vi "hamamatsuRead.vi"   [LabVIEW 2017]
uses:
  globalDevices.vi
  globalUtilities.vi
types:
  T1 = enum16{"open", "replace", "create", "open or create", "replace or create", "replace or create with confirmation"}
  T2 = enum16{"big-endian, network order", "native, host order", "little-endian"}
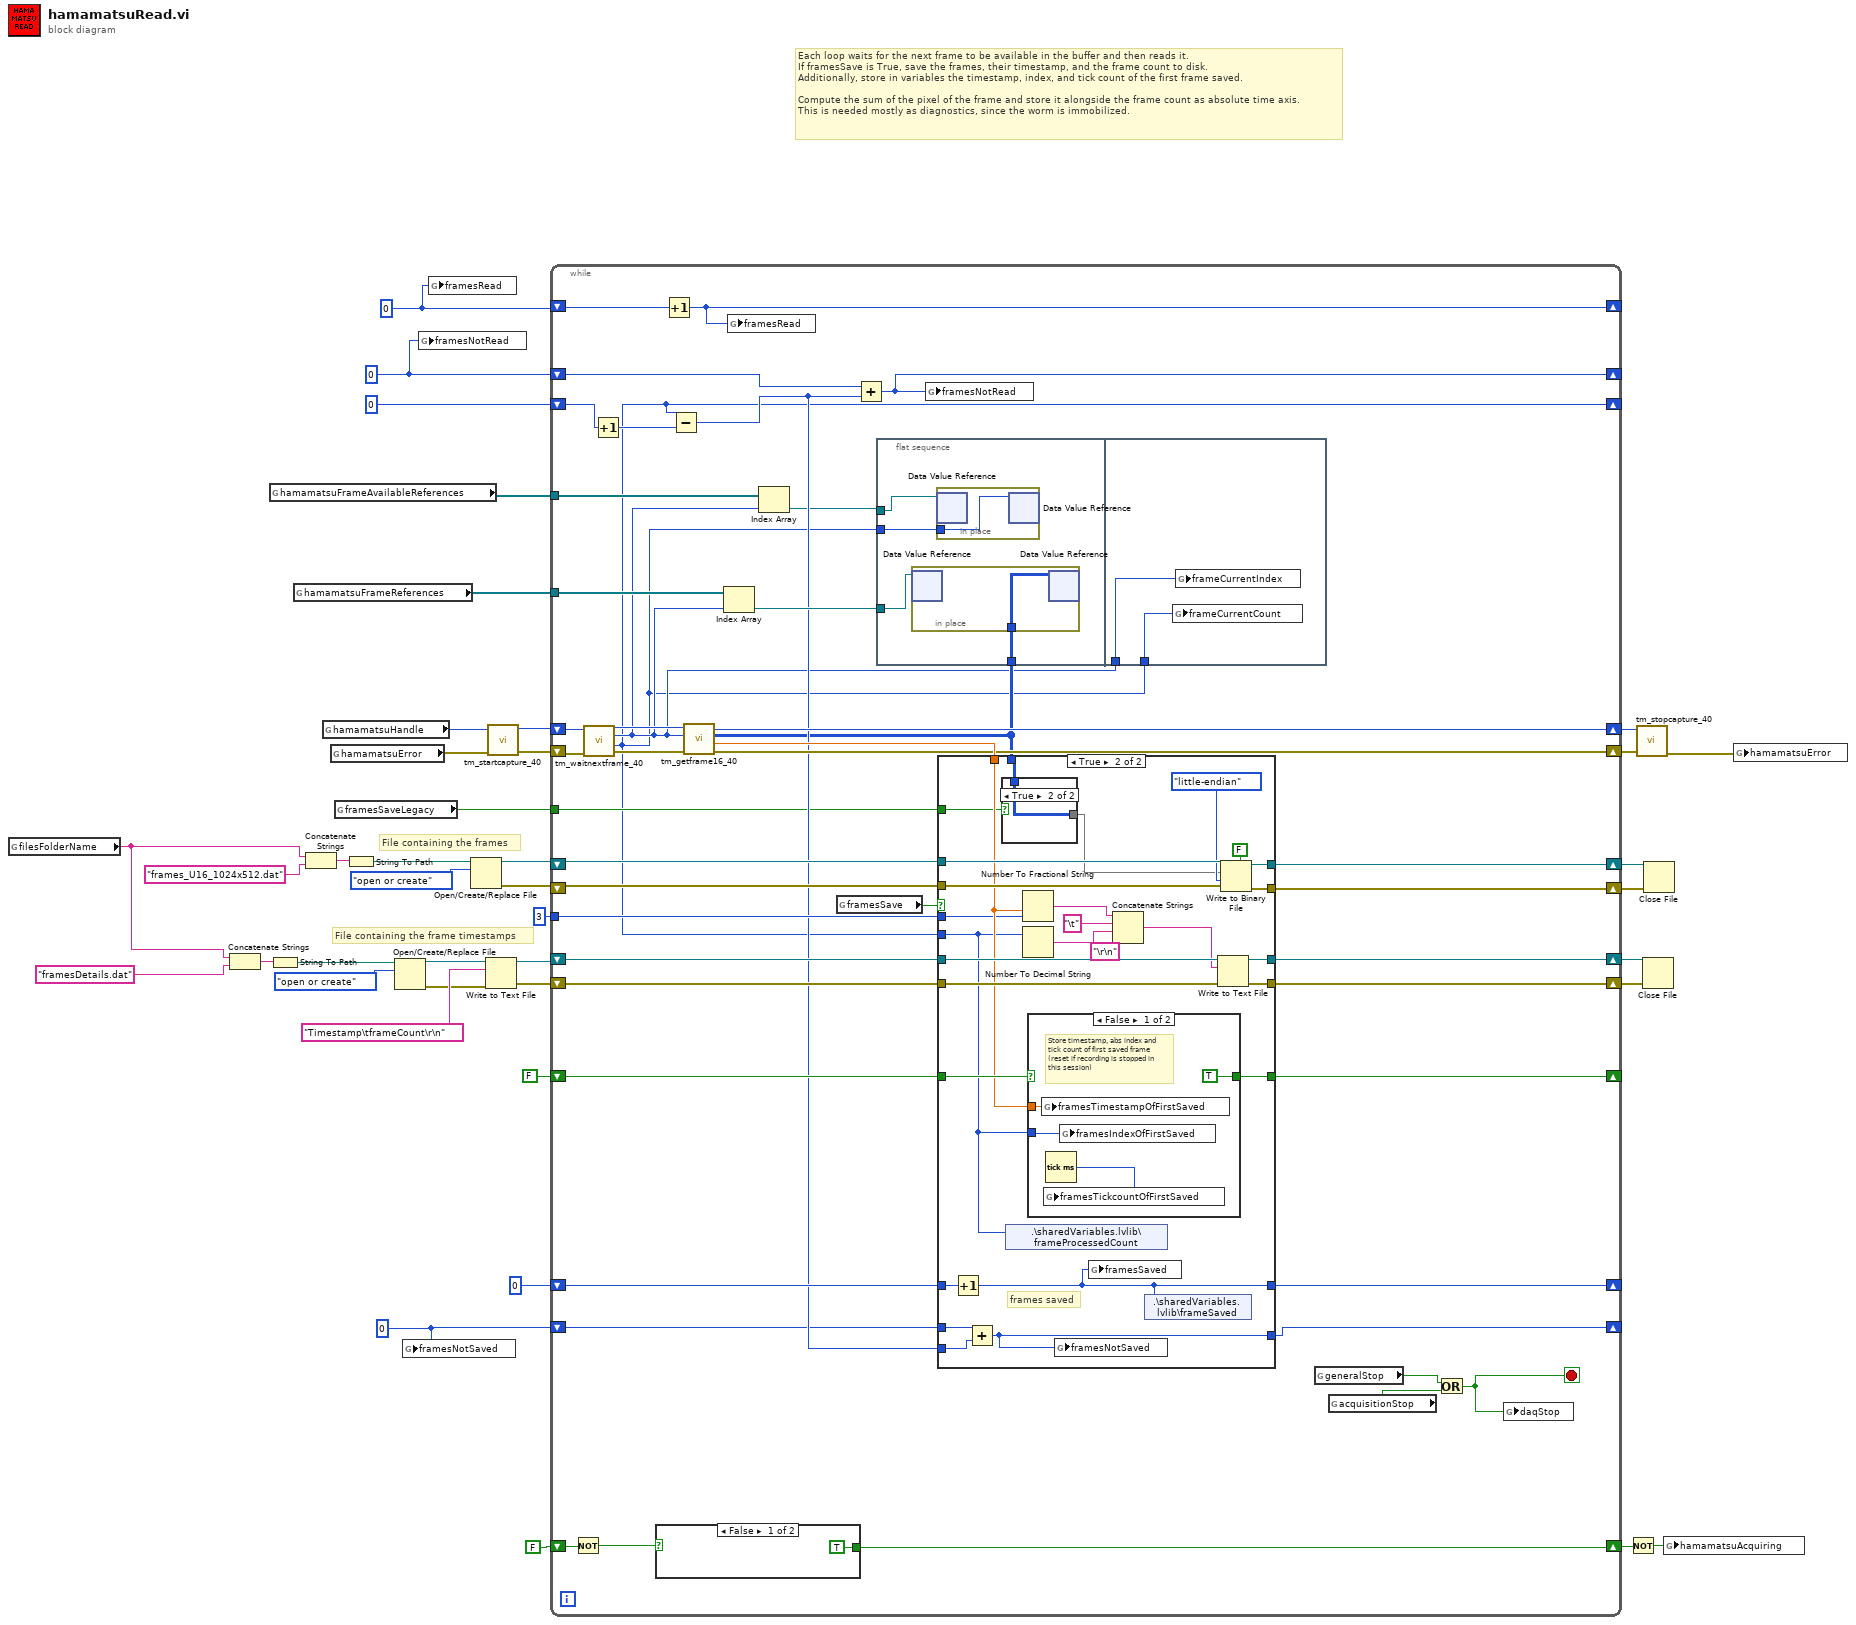
[diagram p0: block diagram]
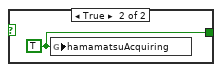
[diagram p2: hidden frame]
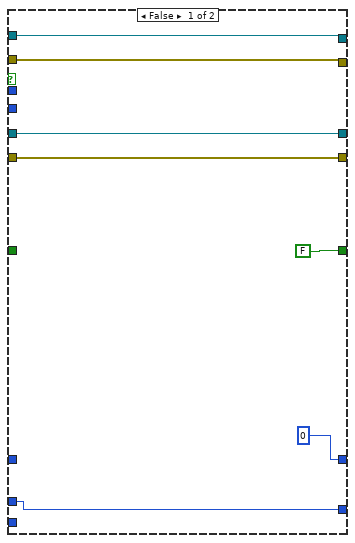
[diagram p3: hidden frame]
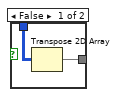
[diagram p4: hidden frame]
diagram:
  w1 = u32 0 ("framesRead")
  w5 = 0
  w2 = 0
  # "Each loop waits for the next frame to be available in the buffer and then reads it.\nIf framesSave is True, save the frames, their timestamp, and the frame count to disk.\nAdditionally, store in variables the timestamp, index, and tick count of the first frame saved.\n\nCompute the sum of the pixel of the frame and store it alongside the frame count as absolute time axis.\nThis is needed mostly as diagnostics, since the worm is immobilized."
  # "File containing the frame timestamps"
  # "File containing the frames"
  n1 = global read "globalUtilities.vi" "filesFolderName"() -> (w23:string)
  n2 = Concatenate Strings(w23, "framesDetails.dat") -> (w33:string)
  n3 = global read "globalDevices.vi" "hamamatsuFrameAvailableReferences"() -> (w6:refnum<data-value>[])
  n4 = String To Path(string=w33) -> (path=w34:path)
  n5 = global read "globalDevices.vi" "hamamatsuFrameReferences"() -> (w10:refnum<data-value>[])
  n6 = Concatenate Strings(w23, "frames_U16_1024x512.dat") -> (w38:string)
  n7 = global read "globalDevices.vi" "hamamatsuHandle"() -> (w19:u32)
  n8 = global read "globalDevices.vi" "hamamatsuError"() -> (w20:errorcluster)
  n9 = global read "globalUtilities.vi" "framesSaveLegacy"() -> (w7:bool)
  n10 = String To Path(string=w38) -> (path=w37:path)
  n11 = Open/Create/Replace File(file path (use dialog)=w34, operation (0:open)=T1."open or create") -> (refnum out=w28:refnum<file>, error out=w26:errorcluster)  [unwired: 4 in, 1 out]
  n12 = global write "globalUtilities.vi" "framesNotSaved"(w5) -> ()
  n13 = global write "globalUtilities.vi" "framesNotRead"(w2) -> ()
  n14 = global write "globalUtilities.vi" "framesRead"(w1) -> ()
  n15 = Open/Create/Replace File(file path (use dialog)=w37, operation (0:open)=T1."open or create") -> (refnum out=w36:refnum<file>, error out=w30:errorcluster)  [unwired: 4 in, 1 out]
  n16 = Write to Text File(file (use dialog)=w28, text="Timestamp\tframeCount\r\n", error in=w26) -> (refnum out=w25:refnum<file>, error out=w24:errorcluster)  [unwired: 1 in, 1 out]
  n17 = call <userlib>:"tm_startcapture_40.vi"("error in (no error)"=w20, "Handle in"=w19) -> ("error out"=w21:errorcluster, "Handle out"=w22:u32)  [unwired: 8 in]
  n18 = while {
    shift-right: [w71] -> _
    shift-left: FALSE -> [w72]
    shift-right: [w77] -> w13
    shift-left: w24 -> [w78]
    shift-right: [w75] -> w15
    shift-left: w30 -> [w76]
    tunnel: i16 3 ("precision (6)") -> [w70]
    shift-right: [w69] -> w18
    shift-left: w21 -> [w83]
    shift-right: [w67] -> _
    shift-left: u32 0 -> [w68]
    shift-right: [w66] -> w17
    shift-left: w22 -> [w84]
    shift-right: [w64] -> w12
    shift-left: w25 -> [w79]
    shift-right: [w65] -> w14
    shift-left: w36 -> [w80]
    tunnel: w10 -> [w60]
    shift-right: [w43] -> _
    shift-left: 0 -> [w58]
    shift-right: [w56] -> _
    shift-left: w2 -> [w57]
    shift-right: [w53] -> _
    shift-left: w5 -> [w54]
    tunnel: w7 -> [w52]
    tunnel: w6 -> [w48]
    shift-right: [w45] -> w3
    shift-left: FALSE -> [w47]
    shift-right: [w41] -> _
    shift-left: w1 -> [w42]
    stop <- w61 stop-if-true
    n19 = Not(x=w47) -> (.not. x?=w46:bool)
    n20 = call <userlib>:"tm_waitnextframe_40.vi"("error in (no error)"=w83, "Handle in"=w84) -> ("error out"=w82:errorcluster, "Frame Count"=w43:i32, "Frame Index"=w49:i32, "Handle out"=w81:u32)  [unwired: 6 in]
    n21 = Increment(x=w58) -> (x+1=w51:i32)
    n22 = case shown="False" w46 {
      tunnel: [TRUE w86] -> w45
      frame False {
      }
      frame True {
        w86 = TRUE ("hamamatsuAcquiring")
        n23 = global write "globalUtilities.vi" "hamamatsuAcquiring"(w86) -> ()
      }
    }
    n24 = Increment(x=w42) -> (x+1=w41:u32)
    n25 = Subtract(x=w43, y=w51) -> (x-y=w55:i32)
    n26 = call <userlib>:"tm_getframe16_40.vi"("error in (no error)"=w82, "Frame Index"=w49, "Handle in"=w81) -> ("error out"=w69:errorcluster, "Timestamp"=w73:dbl, "Data"=w50:u16[][], "Handle out"=w66:u32)  [unwired: 5 in]
    n27 = Index Array(array=w60, index=w49) -> (element=w59:refnum<data-value>)
    n28 = global write "globalUtilities.vi" "framesRead"(w41) -> ()
    n29 = Index Array(array=w48, index=w49) -> (element=w44:refnum<data-value>)
    n30 = global read "globalUtilities.vi" "framesSave"() -> (w74:bool)
    n31 = Add(x=w57, y=w55) -> (x+y=w56:i32)
    n32 = flat-sequence {
      tunnel: w59 -> [w90]
      tunnel: w50 -> [w89]
      tunnel: w44 -> [w88]
      tunnel: w43 -> [w87]
      tunnel: w49 -> [w94]
      tunnel: w43 -> [w93]
      frame #0 {
        n33 = in-place {
          in-place-border: w89 -> [w92]
          n34 = in-place-dvr #1(w90) -> ()  [unwired: 2 out]
          n35 = in-place-dvr #1(w92) -> ()  [unwired: 2 out]
        }
        n36 = in-place {
          in-place-border: w87 -> [w91]
          n37 = in-place-dvr #2(w88) -> ()  [unwired: 2 out]
          n38 = in-place-dvr #2(w91) -> ()  [unwired: 2 out]
        }
      }
      frame #1 {
        n39 = global write "globalUtilities.vi" "frameCurrentCount"(w93) -> ()
        n40 = global write "globalUtilities.vi" "frameCurrentIndex"(w94) -> ()
      }
    }
    n41 = global write "globalUtilities.vi" "framesNotRead"(w56) -> ()
    n42 = case shown="True" w74 {
      tunnel: w80 -> [w97 w129]
      tunnel: w50 -> [_ w105]
      tunnel: w79 -> [w96 w126]
      tunnel: w73 -> [_ w119]
      tunnel: w78 -> [w100 w125]
      tunnel: [w100 w124] -> w77
      tunnel: w76 -> [w101 w123]
      tunnel: [w101 w122] -> w75
      tunnel: w72 -> [_ w121]
      tunnel: [FALSE w120] -> w71
      tunnel: w43 -> [_ w110]
      tunnel: w70 -> [_ w118]
      tunnel: w68 -> [_ w113]
      tunnel: [u32 0 w102] -> w67
      tunnel: [w97 w112] -> w65
      tunnel: [w96 w111] -> w64
      tunnel: w55 -> [_ w108]
      tunnel: w54 -> [w95 w109]
      tunnel: [w95 w107] -> w53
      tunnel: w52 -> [_ w106]
      frame False {
      }
      frame True {
        # "frames saved"
        n43 = Increment(x=w113) -> (x+1=w102:u32)
        n44 = Add(x=w109, y=w108) -> (x+y=w107:i32)
        n45 = case shown="True" w106 {
          tunnel: w105 -> [w131 w132]
          tunnel: [w130 w132] -> w103
          frame False {
            n46 = Transpose 2D Array(2D array=w131) -> (transposed array=w130:u16[][])
          }
          frame True {
          }
        }
        n47 = shared-variable ".\\sharedVariables.lvlib\\frameProcessedCount"(w110) -> ()  [unwired: 1 in, 1 out]
        n48 = Number To Fractional String(number=w119, precision (6)=w118) -> (F-format string=w116:string)  [unwired: 2 in]
        n49 = Number To Decimal String(number=w110) -> (decimal integer string=w115:string)  [unwired: 1 in]
        n50 = case shown="False" w121 {
          selector: w121 -> [_ w137]
          tunnel: [TRUE w137] -> w120
          tunnel: w119 -> [w135 _]
          tunnel: w110 -> [w134 _]
          frame False {
            # "Store timestamp, abs index and\ntick count of first saved frame\n(reset if recording is stopped in\nthis session)"
            n51 = global write "globalUtilities.vi" "framesTimestampOfFirstSaved"(w135) -> ()
            n52 = Tick Count (ms)() -> (millisecond timer value=w133:u32)
            n53 = global write "globalUtilities.vi" "framesTickcountOfFirstSaved"(w133) -> ()
            n54 = global write "globalUtilities.vi" "framesIndexOfFirstSaved"(w134) -> ()
          }
          frame True {
          }
        }
        n55 = global write "globalUtilities.vi" "framesNotSaved"(w107) -> ()
        n56 = global write "globalUtilities.vi" "framesSaved"(w102) -> ()
        n57 = Concatenate Strings(w116, "\t", w115, "\r\n" ("string")) -> (w114:string)
        n58 = shared-variable ".\\sharedVariables.lvlib\\frameSaved"(w102) -> ()  [unwired: 1 in, 1 out]
        n59 = Write to Text File(file (use dialog)=w126, text=w114, error in=w125) -> (refnum out=w111:refnum<file>, error out=w124:errorcluster)  [unwired: 1 in, 1 out]
        n60 = Write to Binary File(file (use dialog)=w129, data=w103, error in=w123, 5:FALSE ("prepend array or string size? (T)"), 9:T2."little-endian" ("byte order (0:big-endian, network order)")) -> (refnum out=w112:refnum<file>, error out=w122:errorcluster)  [unwired: 1 in, 1 out]
      }
    }
    n61 = global read "globalUtilities.vi" "generalStop"() -> (w63:bool)
    n62 = global read "globalUtilities.vi" "acquisitionStop"() -> (w62:bool)
    n63 = Or(x=w63, y=w62) -> (x .or. y?=w61:bool)
    n64 = global write "globalUtilities.vi" "daqStop"(w61) -> ()
  }
  n65 = Not(x=w3) -> (.not. x?=w11:bool)
  n66 = call <userlib>:"tm_stopcapture_40.vi"("error in (no error)"=w18, "Handle in"=w17) -> ("error out"=w16:errorcluster)  [unwired: 8 in, 1 out]
  n67 = Close File(refnum=w12, error in=w13) -> ()  [unwired: 2 out]
  n68 = Close File(refnum=w14, error in=w15) -> ()  [unwired: 2 out]
  n69 = global write "globalUtilities.vi" "hamamatsuAcquiring"(w11) -> ()
  n70 = global write "globalDevices.vi" "hamamatsuError"(w16) -> ()
